vi "reward_behavior_timeout_9s_probes_opto_2-5s_ISI.vi"() -> ()   [LabVIEW 2019]
doc: "The myRIO Project template acquires acceleration data from the onboard accelerometer and displays the changes of acceleration values in a waveform chart."
uses:
  <vilib>/Analysis/Matrix/Datatypes/RealMatrix.ctl
  <vilib>/myRIO/Common/Instrument Driver Framework/myRIO v1.0/Encoder/typedefs/Encoder Signal Mode.ctl
  <vilib>/myRIO/Instrument Drivers/Onboard IO/Encoder/typedefs/Encoder Reference.ctl
  <vilib>/myRIO/Common/Instrument Driver Framework/Utilities/typedefs/myRIO Generic Hardware Reference.ctl
  <vilib>/myRIO/Common/Instrument Driver Framework/Utilities/typedefs/Hardware Version Enum.ctl
  <vilib>/myRIO/Common/Instrument Driver Framework/Utilities/typedefs/myRIO v1.0 Reference.ctl
  <vilib>/myRIO/Common/Instrument Driver Framework/Utilities/typedefs/Generic FPGA Reference.ctl
  <vilib>/myRIO/Common/Instrument Driver Framework/myRIO v1.0/Encoder/typedefs/Encoder Channels Enum.ctl
  <vilib>/myRIO/Common/Instrument Driver Framework/myRIO v1.0/Encoder/typedefs/Encoder Configuration v1.0.ctl
  <vilib>/userdefined/High Color/nirio_resource_hc.ctl
  <vilib>/myRIO/Instrument Drivers/Onboard IO/DIO/typedefs/DIO Reference.ctl
  <vilib>/myRIO/Common/Instrument Driver Framework/myRIO v1.0/DIO/typedefs/DIO Channels List.ctl
  <vilib>/myRIO/Common/Instrument Driver Framework/myRIO v1.0/DIO/typedefs/DIO Channels Enum.ctl
  <vilib>/myRIO/Common/Instrument Driver Framework/Utilities/vis/Is FPGA Ref Available.vi
  <vilib>/myRIO/Common/Instrument Driver Framework/myRIO v1.0/Encoder/vis/myRIO v1.1 Open Encoder.vi
  <vilib>/myRIO/Instrument Drivers/Onboard IO/Encoder/vis/Read.vi
  <vilib>/myRIO/Common/Instrument Driver Framework/myRIO v1.0/DIO/vis/myRIO v1.1 Open DIO.vi
  <vilib>/myRIO/Instrument Drivers/Onboard IO/DIO/vis/Write.vi
  <vilib>/myRIO/Instrument Drivers/Onboard IO/DIO/vis/Read.vi
  <vilib>/myRIO/Common/Instrument Driver Framework/Utilities/vis/Validate Channels.vi
  <vilib>/myRIO/Common/Instrument Driver Framework/myRIO v1.0/Encoder/vis/myRIO v1.0 Reserve Encoder.vi
  <vilib>/myRIO/Common/Instrument Driver Framework/myRIO v1.0/DIO/vis/myRIO v1.0 Reserve DIO.vi
  <vilib>/myRIO/Common/Instrument Driver Framework/myRIO v1.0/Encoder/vis/myRIO v1.0 Build MUX Configuration Encoder.vi
  <vilib>/myRIO/Common/Instrument Driver Framework/myRIO v1.0/Resource Manager/vis/myRIO v1.0 Reserve Channel List.vi
  <vilib>/myRIO/Common/Instrument Driver Framework/myRIO v1.0/DIO/vis/myRIO v1.0 Build MUX Configuration DIO.vi
  <vilib>/myRIO/Common/Instrument Driver Framework/myRIO v1.0/Resource Manager/vis/myRIO v1.0 Create Configuration List.vi
  <vilib>/myRIO/Common/Instrument Driver Framework/myRIO v1.0/Resource Manager/vis/myRIO v1.0 Reserve Channel.vi
  <vilib>/myRIO/Common/Instrument Driver Framework/myRIO v1.0/Resource Manager/vis/myRIO v1.0 Unreserve Channel.vi
  <vilib>/myRIO/Common/Instrument Driver Framework/myRIO v1.0/Resource Manager/vis/myRIO v1.0 Build Mutex Name.vi
  <vilib>/Utility/VariantDataType/GetNumericInfo.vi
  <vilib>/Utility/error.llb/Error Cluster From Error Code.vi
  <vilib>/myRIO/Common/Instrument Driver Framework/myRIO v1.0/myRIO v1.1 Open.vi
  <vilib>/myRIO/Common/Instrument Driver Framework/Utilities/vis/IO Manager.vi
  <vilib>/myRIO/Common/Instrument Driver Framework/Utilities/vis/Configuration Manager.vi
  <vilib>/myRIO/Common/Instrument Driver Framework/myRIO v1.0/Resource Manager/vis/myRIO v1.0 Configure IO.vi
  <vilib>/myRIO/Common/Instrument Driver Framework/myRIO v1.0/myRIO v1.0 Close.vi
  <vilib>/myRIO/Common/Instrument Driver Framework/myRIO v1.0/Encoder/vis/myRIO v1.0 Configure Encoder.vi
  <vilib>/myRIO/Common/Instrument Driver Framework/myRIO v1.0/Encoder/vis/myRIO v1.0 Read Encoder.vi
  <vilib>/myRIO/Common/Instrument Driver Framework/myRIO v1.0/DIO/vis/myRIO v1.0 Read DIO.vi
  <vilib>/myRIO/Common/Instrument Driver Framework/myRIO v1.0/DIO/vis/myRIO v1.0 Write DIO.vi
  <vilib>/myRIO/Express VI/Onboard IO/Encoder/Encoder Express VI.xnode
  <vilib>/myRIO/Instrument Drivers/Onboard IO/Encoder/vis/myRIO Encoder Open.xnode
  <vilib>/myRIO/Express VI/Onboard IO/DI/DI Express VI.xnode
  <vilib>/myRIO/Instrument Drivers/Onboard IO/DIO/vis/myRIO DIO Open.xnode
  <vilib>/myRIO/Express VI/Onboard IO/DO/DO Express VI.xnode
  <vilib>/myRIO/Instrument Drivers/Onboard IO/Encoder/Encoder.lvlib
  <vilib>/myRIO/Instrument Drivers/Onboard IO/DIO/DIO.lvlib
  <vilib>/Analysis/Matrix/NI_Matrix.lvlib
panel:
  out "Timings":dbl[](array[numeric])
  out "ISI":dbl
  out "ISI start time":dbl
  out "Time_out":bool=TRUE
  out "Time since lick":dbl
  out "Time of last lick":dbl
  out "Rewarded trials":dbl[](array[numeric])
  out "Rewards":u16
  out "Active Trial":bool
  out "Array temp2":T1
  out "Stimuli Loaded":bool
  out "Stim_ID":dbl[](array[numeric])
  out "Reward_mat":dbl[](array[numeric])
  out "Reward":bool=TRUE
  out "Frame clock":i32
  out "Licks":u32
  out "Lick":bool
  out "Time":dbl
  out "Stop":bool
  in  "Frames to collect":u32
  out "Overflow?":bool
  out "Counter Value":i32
  out "Velocity":dbl
  out "Velocity Plot":dbl[](graph)
  out "Velocity array":dbl[](array[numeric])
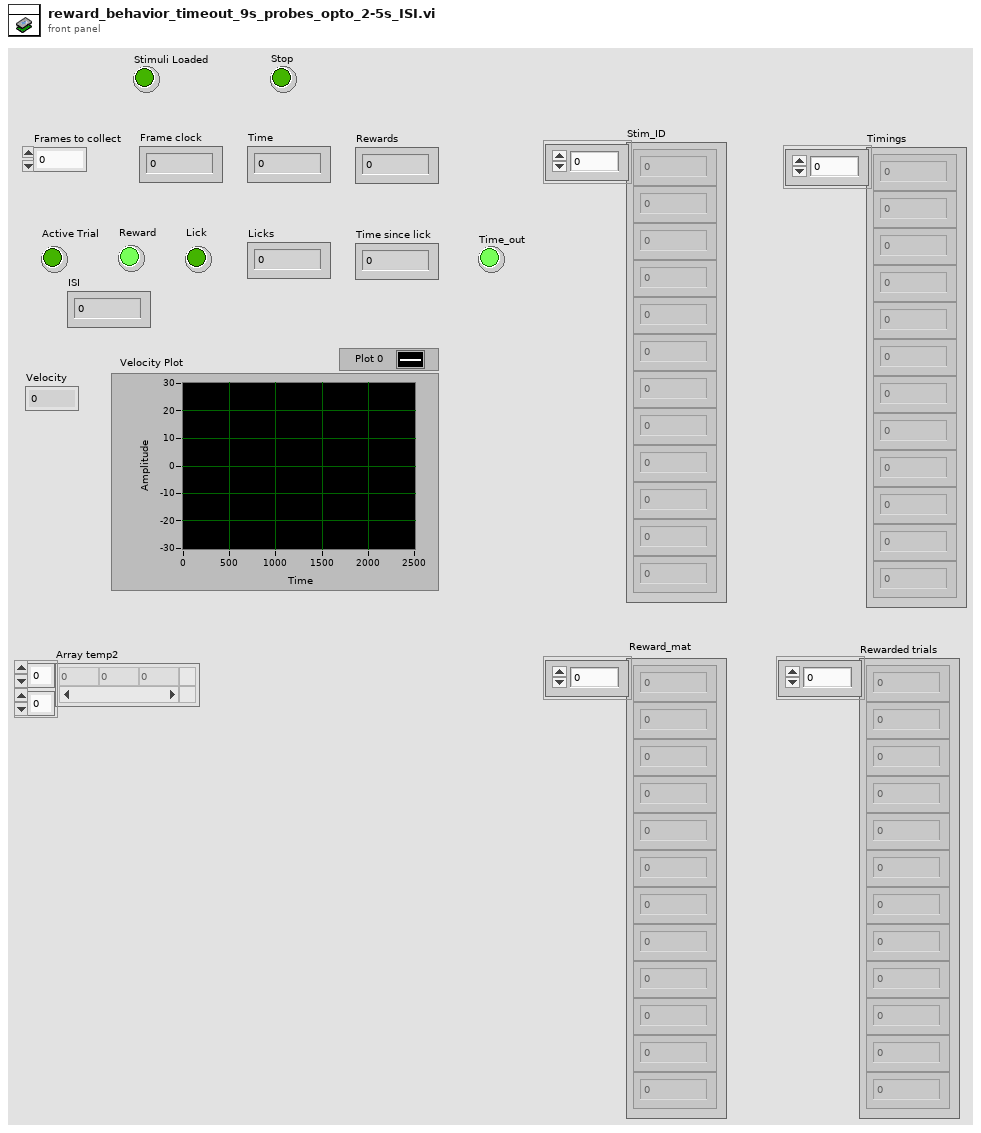
[diagram p1: front panel]
types:
  T1 = typedef "NI_Matrix.lvlib/RealMatrix.ctl" = dbl[][]
  T2 = typedef "Encoder.lvlib/Encoder Reference.ctl" = cluster{"myRIO Reference":T3, "Encoder Channels Enum":T7}
  T3 = typedef "myRIO Generic Hardware Reference.ctl" = cluster{"myRIO Model":T4, "myRIO Hardware Reference":T5}
  T4 = typedef "Hardware Version Enum.ctl" = enum16{"Unknown", "myRIO-1900", "myRIO-1950", "roboRIO", "NI ELVIS RIO CM", "ELVIS III"}
  T5 = typedef "myRIO v1.0 Reference.ctl" = cluster{"Generic FPGA Reference":T6, "Allow multiple opens":bool}
  T6 = typedef "Generic FPGA Reference.ctl" = refnum<k20>
  T7 = typedef "Encoder Channels Enum.ctl" = enum16{"Not Connected", "C/ENC0", "C/ENC1", "A/ENC", "A/ENC0", "A/ENC1", "A/ENC2", "A/ENC3", "A/ENC4", "A/ENC5", "A/ENC6", "A/ENC7", "A/ENC8", "A/ENC9", "B/ENC", "B/ENC0", "B/ENC1", "B/ENC2", "B/ENC3", "B/ENC4", "B/ENC5", "B/ENC6", "B/ENC7", "B/ENC8", "B/ENC9", "DIO/ENC0", "DIO/ENC1", "DIO/ENC2", "DIO/ENC3", "DIO/ENC4"}
  T8 = typedef "Encoder Signal Mode.ctl" = enum16{"Quadrature phase signal", "Step and direction signal"}
  T9 = typedef "nirio_resource_hc.ctl" = tag
  T10 = typedef "DIO.lvlib/DIO Reference.ctl" = cluster{"myRIO Reference":T3, "DIO Channels List":T11}
  T11 = typedef "DIO Channels List.ctl" = T12[]
  T12 = typedef "DIO Channels Enum.ctl" = enum16{"Not Connected", "C/DIO0", "C/DIO1", "C/DIO2", "C/DIO3", "C/DIO4", "C/DIO5", "C/DIO6", "C/DIO7", "A/DIO0", "A/DIO1", "A/DIO2", "A/DIO3", "A/DIO4", "A/DIO5", "A/DIO6", "A/DIO7", "A/DIO8", "A/DIO9", "A/DIO10", "A/DIO11", "A/DIO12", "A/DIO13", "A/DIO14", "A/DIO15", "A/DIO16", "A/DIO17", "A/DIO18", "A/DIO19", "B/DIO0", "B/DIO1", "B/DIO2", "B/DIO3", "B/DIO4", "B/DIO5", "B/DIO6", "B/DIO7", "B/DIO8", "B/DIO9", "B/DIO10", "B/DIO11", "B/DIO12", "B/DIO13", "B/DIO14", "B/DIO15", "B/DIO16", "B/DIO17", "B/DIO18", "B/DIO19", "LED0", "LED1", "LED2", "LED3", "Button0", "DIO/DIO0", "DIO/DIO1", "DIO/DIO2", "DIO/DIO3", "DIO/DIO4", "DIO/DIO5", "DIO/DIO6", "DIO/DIO7", "DIO/DIO8", "DIO/DIO9", "SPI/CS0", "SPI/CS1", "SPI/CS2", "SPI/CS3", "LED RADIO (Green)", "LED RADIO (Red)", "LED COMM (Green)", "LED COMM (Red)", "LED MODE (Green)", "LED MODE (Red)"}
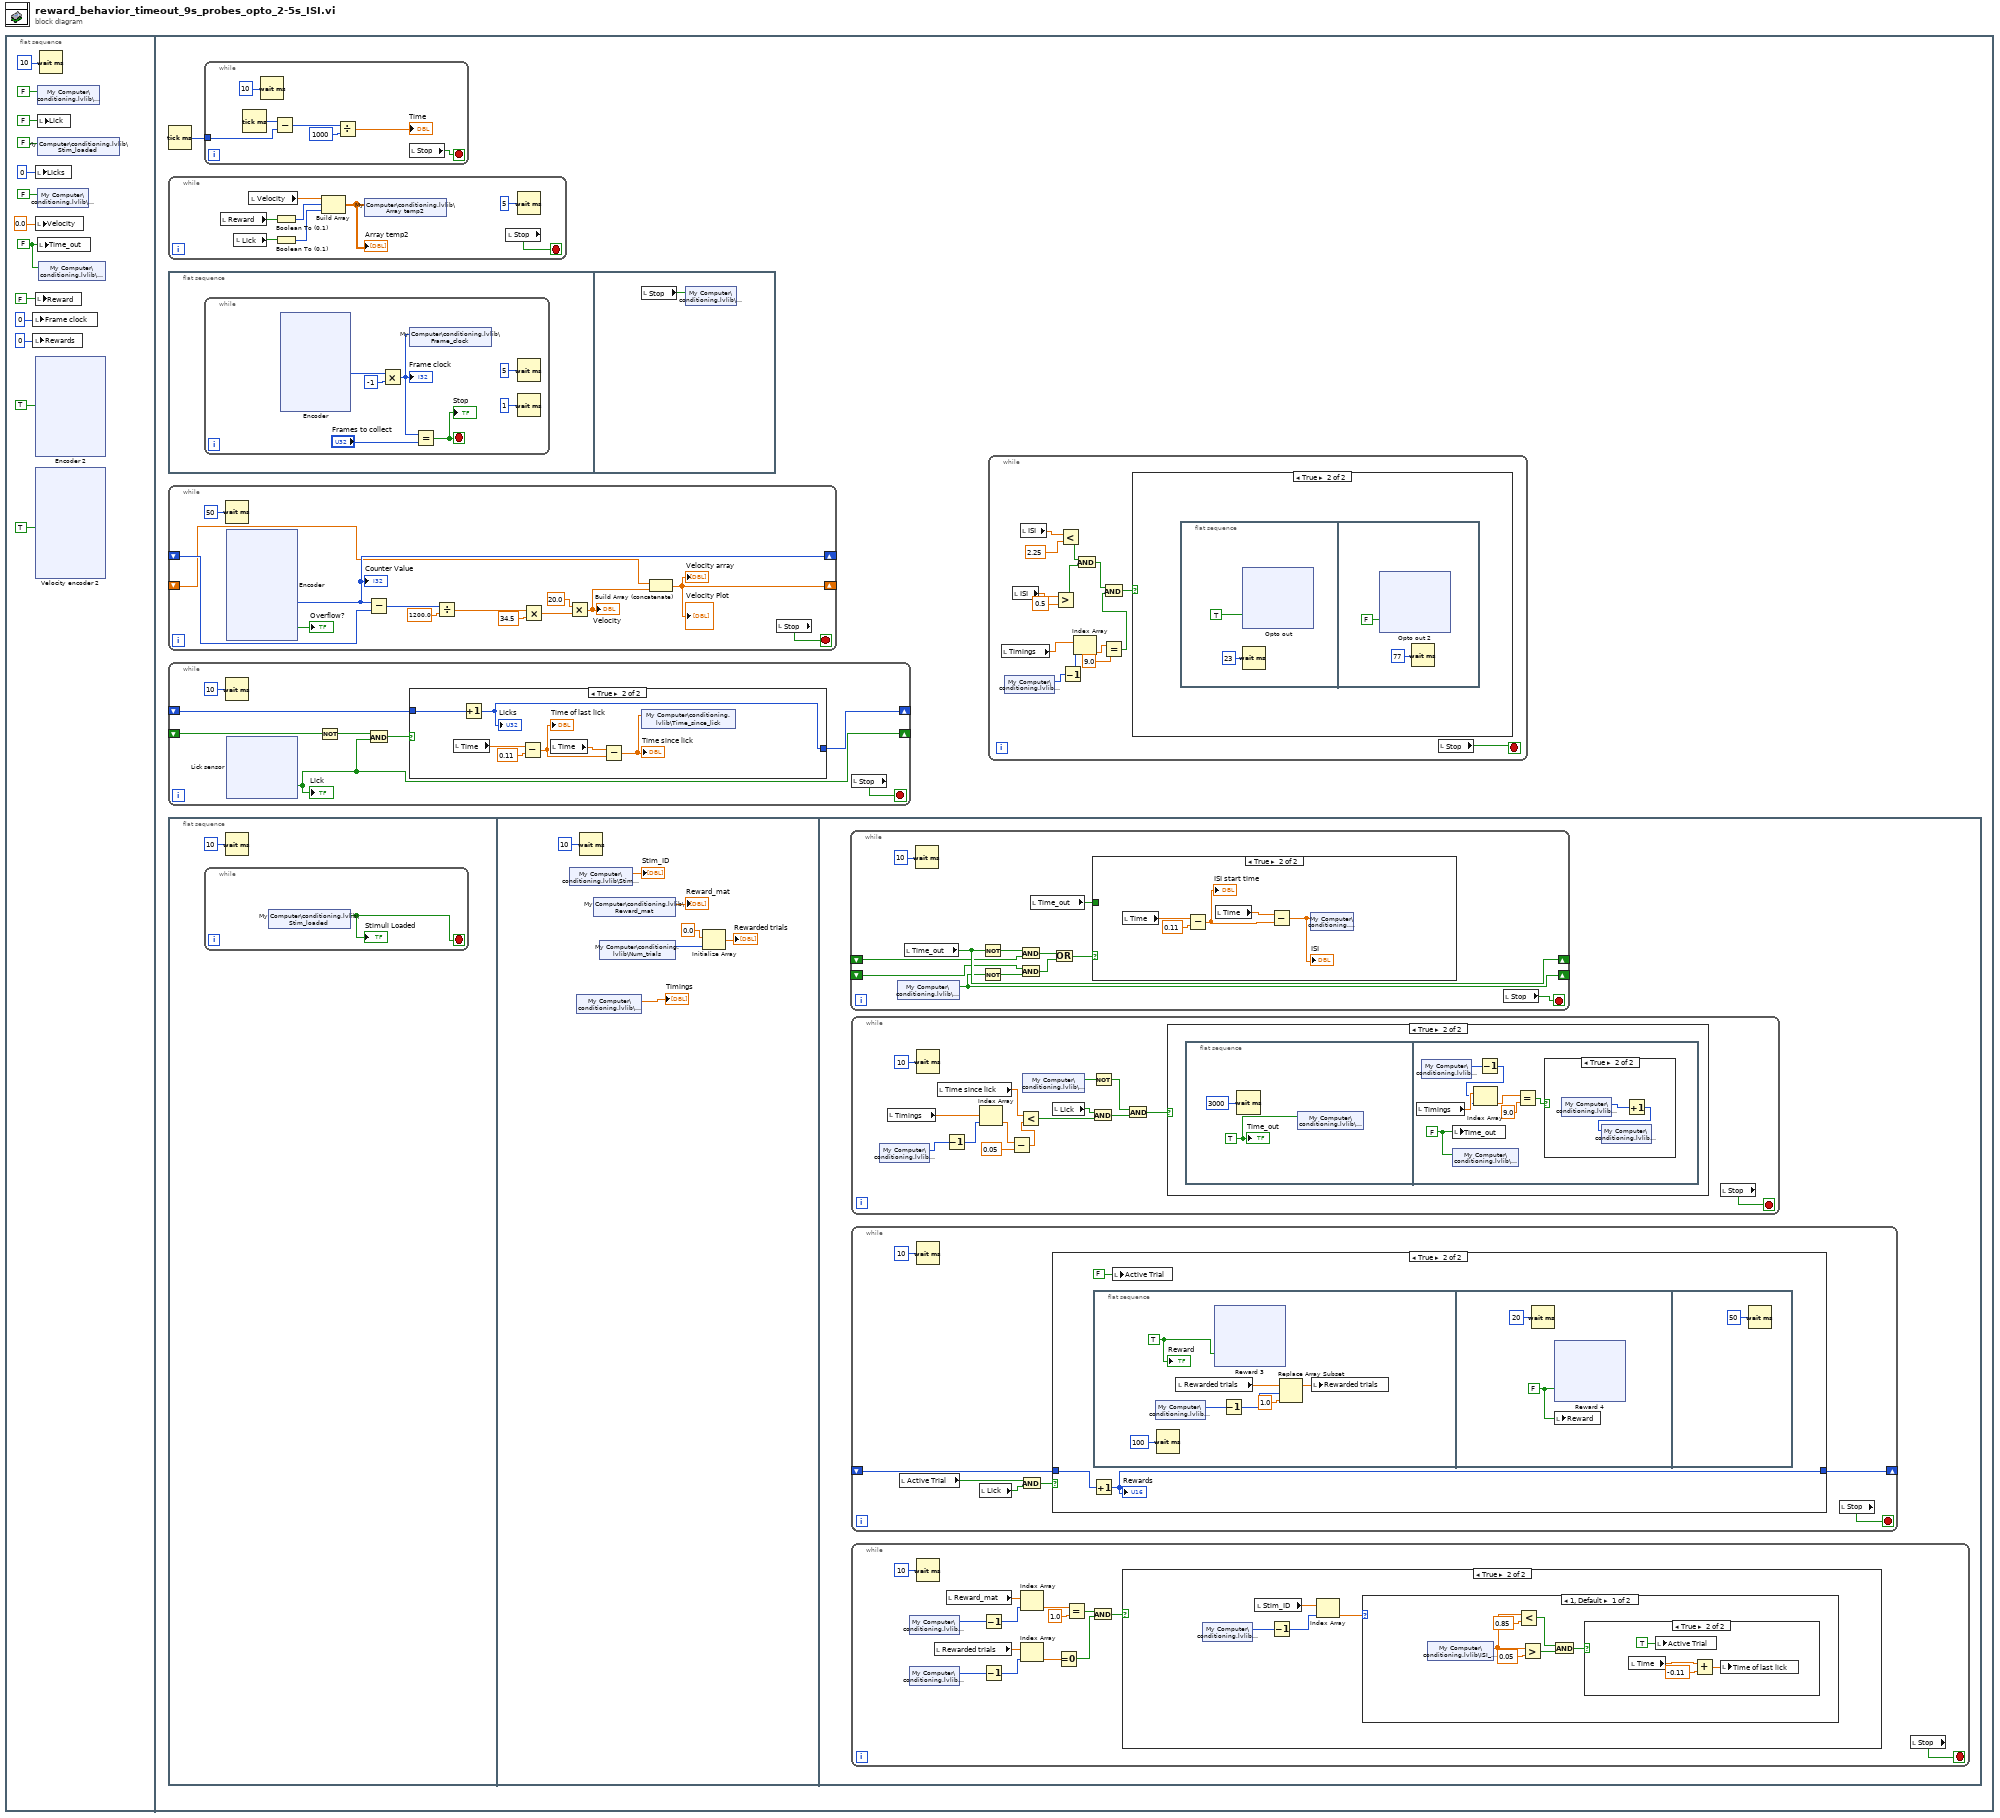
[diagram p0: block diagram]
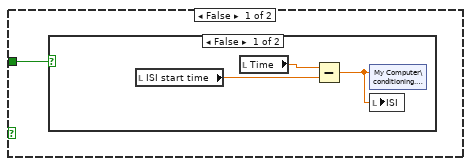
[diagram p5: hidden frame]
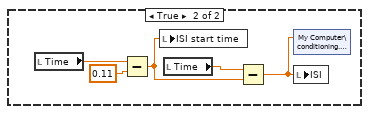
[diagram p6: hidden frame]
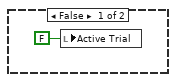
[diagram p7: hidden frame]
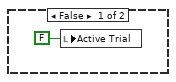
[diagram p8: hidden frame]
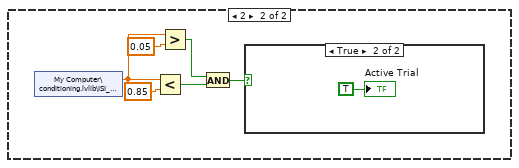
[diagram p9: hidden frame]
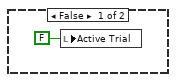
[diagram p10: hidden frame]
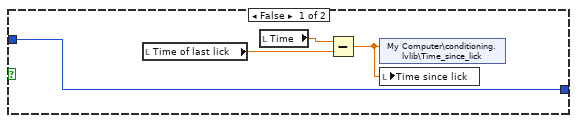
[diagram p12: hidden frame]
diagram:
  n1 = flat-sequence {
    frame #0 {
      w1 = FALSE ("Time_out")
      n2 = local write "Frame clock"(u32 0 ("Frames")) -> ()
      n3 = local write "Rewards"(u16 0 ("Rewards")) -> ()
      n4 = local write "Licks"(u32 0 ("Licks")) -> ()
      n5 = local write "Velocity"(0.0 ("Velocity")) -> ()
      n6 = local write "Reward"(FALSE ("Give reward")) -> ()
      n7 = xnode "Encoder 2"("Reset Counter"=TRUE) -> ()  [unwired: 1 in, 4 out]
      n8 = xnode "Velocity encoder 2"("Reset Counter"=TRUE) -> ()  [unwired: 1 in, 4 out]
      n9 = shared-variable "My Computer\\conditioning.lvlib\\Display"(FALSE ("Display")) -> ()  [unwired: 1 in, 1 out]
      n10 = local write "Lick"(FALSE ("Lick")) -> ()
      n11 = shared-variable "My Computer\\conditioning.lvlib\\Stim_loaded"(FALSE ("Stim_loaded")) -> ()  [unwired: 1 in, 1 out]
      n12 = shared-variable "My Computer\\conditioning.lvlib\\Stop"(FALSE ("Stop")) -> ()  [unwired: 1 in, 1 out]
      n13 = local write "Time_out"(w1) -> ()
      n14 = shared-variable "My Computer\\conditioning.lvlib\\Timeout"(w1) -> ()  [unwired: 1 in, 1 out]
      n15 = Wait (ms)(milliseconds to wait=u32 10) -> ()  [unwired: 1 out]
    }
    frame #1 {
      n16 = Tick Count (ms)() -> (millisecond timer value=w106:u32)
      n17 = while {
        stop <- w197 stop-if-true
        n18 = local read "Reward"() -> (w202:bool)
        n19 = local read "Lick"() -> (w203:bool)
        n20 = local read "Velocity"() -> (w201:dbl)
        n21 = Boolean To (0,1)(Boolean=w202) -> (0, 1=w200:i16)
        n22 = Boolean To (0,1)(Boolean=w203) -> (0, 1=w199:i16)
        n23 = Build Array(w201, w200, w199) -> (w196:T1)
        "Array temp2" <- w196
        n24 = shared-variable "My Computer\\conditioning.lvlib\\Array temp2"(w196) -> ()  [unwired: 1 in, 1 out]
        n25 = local read "Stop"() -> (w197:bool)
        n26 = Wait (ms)(milliseconds to wait=u32 5) -> ()  [unwired: 1 out]
      }
      n27 = flat-sequence {
        frame #0 {
          n28 = while {
            stop <- w395 stop-if-true
            n29 = xnode "Encoder"() -> ("Counter Value"=w399:i32)  [unwired: 2 in, 3 out]
            n30 = Multiply(x=w399, y=-1) -> (x*y=w394:i32)
            "Frame clock" <- w394
            n31 = shared-variable "My Computer\\conditioning.lvlib\\Frame_clock"(w394) -> ()  [unwired: 1 in, 1 out]
            n32 = Equal?(x=w394, y="Frames to collect") -> (x = y?=w395:bool)
            "Stop" <- w395
            n33 = Wait (ms)(milliseconds to wait=u32 5) -> ()  [unwired: 1 out]
            n34 = Wait (ms)(milliseconds to wait=u32 1) -> ()  [unwired: 1 out]
          }
        }
        frame #1 {
          n35 = local read "Stop"() -> (w447:bool)
          n36 = shared-variable "My Computer\\conditioning.lvlib\\Stop"(w447) -> ()  [unwired: 1 in, 1 out]
        }
      }
      n37 = while {
        shift-right: [w512] -> _
        shift-left: _ -> [w513]
        shift-right: [w504] -> _
        shift-left: _ -> [w503]
        stop <- w502 stop-if-true
        n38 = Wait (ms)(milliseconds to wait=u32 50) -> ()  [unwired: 1 out]
        n39 = xnode "Encoder"() -> ("Counter Value"=w512:i32, "Overflow?"=→"Overflow?":bool)  [unwired: 2 in, 2 out]
        "Counter Value" <- w512
        n40 = Subtract(x=w512, y=w513) -> (x-y=w505:i32)
        n41 = Divide(x=w505, y=1200.0 ("600")) -> (x/y=w510:dbl)
        n42 = Multiply(x=w510, y=34.5) -> (x*y=w508:dbl)
        n43 = Multiply(x=20.0, y=w508) -> (x*y=w506:dbl)
        "Velocity" <- w506
        n44 = Build Array (concatenate)(w503, w506) -> (w504:dbl[])
        "Velocity Plot" <- w504
        "Velocity array" <- w504
        n45 = local read "Stop"() -> (w502:bool)
      }
      n46 = while {
        shift-right: [w454] -> _
        shift-left: _ -> [w453]
        shift-right: [w448] -> _
        shift-left: _ -> [w451]
        stop <- w452 stop-if-true
        n47 = Wait (ms)(milliseconds to wait=u32 10) -> ()  [unwired: 1 out]
        n48 = xnode "Lick sensor"() -> ("C/DIO1 (DIO1)"=w448:bool)  [unwired: 1 in, 1 out]
        "Lick" <- w448
        n49 = Not(x=w451) -> (.not. x?=w450:bool)
        n50 = And(x=w450, y=w448) -> (x .and. y?=w449:bool)
        n51 = case shown="True" w449 {
          tunnel: [w459 w466] -> w454
          tunnel: w453 -> [w459 w465]
          frame False {
            n52 = local read "Time of last lick"() -> (w457:dbl)
            n53 = local read "Time"() -> (w458:dbl)
            n54 = Subtract(x=w458, y=w457) -> (x-y=w456:dbl)
            n55 = shared-variable "My Computer\\conditioning.lvlib\\Time_since_lick"(w456) -> ()  [unwired: 1 in, 1 out]
            n56 = local write "Time since lick"(w456) -> ()
          }
          frame True {
            n57 = local read "Time"() -> (w462:dbl)
            n58 = Increment(x=w465) -> (x+1=w466:u32)
            "Licks" <- w466
            n59 = Subtract(x=w462, y=0.11) -> (x-y=w460:dbl)
            "Time of last lick" <- w460
            n60 = local read "Time"() -> (w464:dbl)
            n61 = Subtract(x=w464, y=w460) -> (x-y=w463:dbl)
            "Time since lick" <- w463
            n62 = shared-variable "My Computer\\conditioning.lvlib\\Time_since_lick"(w463) -> ()  [unwired: 1 in, 1 out]
          }
        }
        n63 = local read "Stop"() -> (w452:bool)
      }
      n64 = flat-sequence {
        frame #0 {
          n65 = while {
            stop <- w205 stop-if-true
            n66 = shared-variable "My Computer\\conditioning.lvlib\\Stim_loaded"() -> (w205:bool)  [unwired: 1 in, 1 out]
            "Stimuli Loaded" <- w205
          }
          n67 = Wait (ms)(milliseconds to wait=u32 10) -> ()  [unwired: 1 out]
        }
        frame #1 {
          n68 = shared-variable "My Computer\\conditioning.lvlib\\Stim_ID"() -> (→"Stim_ID":dbl[])  [unwired: 1 in, 1 out]
          n69 = shared-variable "My Computer\\conditioning.lvlib\\Timings"() -> (→"Timings":dbl[])  [unwired: 1 in, 1 out]
          n70 = Wait (ms)(milliseconds to wait=u32 10) -> ()  [unwired: 1 out]
          n71 = shared-variable "My Computer\\conditioning.lvlib\\Reward_mat"() -> (→"Reward_mat":dbl[])  [unwired: 1 in, 1 out]
          n72 = shared-variable "My Computer\\conditioning.lvlib\\Num_trials"() -> (w209:u32)  [unwired: 1 in, 1 out]
          n73 = Initialize Array(0.0 ("element"), w209) -> (→"Rewarded trials":dbl[])
        }
        frame #2 {
          n74 = while {
            shift-right: [w249] -> _
            shift-left: _ -> [w247]
            shift-right: [w245] -> _
            shift-left: _ -> [w244]
            stop <- w250 stop-if-true
            n75 = shared-variable "My Computer\\conditioning.lvlib\\Display"() -> (w245:bool)  [unwired: 1 in, 1 out]
            n76 = local read "Time_out"() -> (w249:bool)
            n77 = Wait (ms)(milliseconds to wait=u32 10) -> ()  [unwired: 1 out]
            n78 = Not(x=w249) -> (.not. x?=w248:bool)
            n79 = Not(x=w245) -> (.not. x?=w243:bool)
            n80 = And(x=w248, y=w247) -> (x .and. y?=w242:bool)
            n81 = And(x=w244, y=w243) -> (x .and. y?=w241:bool)
            n82 = local read "Time_out"() -> (w246:bool)
            n83 = Or(x=w242, y=w241) -> (x .or. y?=w240:bool)
            n84 = case shown="True" w240 {
              tunnel: w246 -> [w251 _]
              frame False {
                n85 = case shown="False" w251 {
                  frame False {
                    n86 = local read "ISI start time"() -> (w254:dbl)
                    n87 = local read "Time"() -> (w253:dbl)
                    n88 = Subtract(x=w253, y=w254) -> (x-y=w252:dbl)
                    n89 = shared-variable "My Computer\\conditioning.lvlib\\ISI"(w252) -> ()  [unwired: 1 in, 1 out]
                    n90 = local write "ISI"(w252) -> ()
                  }
                  frame True {
                    n91 = local read "Time"() -> (w259:dbl)
                    n92 = Subtract(x=w259, y=0.11) -> (x-y=w256:dbl)
                    n93 = local write "ISI start time"(w256) -> ()
                    n94 = local read "Time"() -> (w257:dbl)
                    n95 = Subtract(x=w257, y=w256) -> (x-y=w255:dbl)
                    n96 = shared-variable "My Computer\\conditioning.lvlib\\ISI"(w255) -> ()  [unwired: 1 in, 1 out]
                    n97 = local write "ISI"(w255) -> ()
                  }
                }
              }
              frame True {
                n98 = local read "Time"() -> (w264:dbl)
                n99 = Subtract(x=w264, y=0.11) -> (x-y=w261:dbl)
                "ISI start time" <- w261
                n100 = local read "Time"() -> (w262:dbl)
                n101 = Subtract(x=w262, y=w261) -> (x-y=w260:dbl)
                "ISI" <- w260
                n102 = shared-variable "My Computer\\conditioning.lvlib\\ISI"(w260) -> ()  [unwired: 1 in, 1 out]
              }
            }
            n103 = local read "Stop"() -> (w250:bool)
          }
          n104 = while {
            stop <- w227 stop-if-true
            n105 = shared-variable "My Computer\\conditioning.lvlib\\Trial"() -> (w217:u32)  [unwired: 1 in, 1 out]
            n106 = local read "Timings"() -> (w218:dbl[])
            n107 = Wait (ms)(milliseconds to wait=u32 10) -> ()  [unwired: 1 out]
            n108 = local read "Time since lick"() -> (w226:dbl)
            n109 = Decrement(x=w217) -> (x-1=w216:u32)
            n110 = Index Array(array=w218, index=w216) -> (element=w215:dbl)
            n111 = Subtract(x=w215, y=0.05) -> (x-y=w213:dbl)
            n112 = Less?(x=w226, y=w213) -> (x < y?=w225:bool)
            n113 = shared-variable "My Computer\\conditioning.lvlib\\Display"() -> (w222:bool)  [unwired: 1 in, 1 out]
            n114 = local read "Lick"() -> (w224:bool)
            n115 = Not(x=w222) -> (.not. x?=w221:bool)
            n116 = And(x=w224, y=w225) -> (x .and. y?=w220:bool)
            n117 = And(x=w221, y=w220) -> (x .and. y?=w219:bool)
            n118 = case shown="True" w219 {
              frame False {
              }
              frame True {
                n119 = flat-sequence {
                  frame #0 {
                    w229 = TRUE
                    n120 = Wait (ms)(milliseconds to wait=u32 3000) -> ()  [unwired: 1 out]
                    n121 = shared-variable "My Computer\\conditioning.lvlib\\Timeout"(w229) -> ()  [unwired: 1 in, 1 out]
                    "Time_out" <- w229
                  }
                  frame #1 {
                    w236 = FALSE ("Timeout")
                    n122 = local read "Timings"() -> (w235:dbl[])
                    n123 = shared-variable "My Computer\\conditioning.lvlib\\Trial"() -> (w231:u32)  [unwired: 1 in, 1 out]
                    n124 = local write "Time_out"(w236) -> ()
                    n125 = shared-variable "My Computer\\conditioning.lvlib\\Timeout"(w236) -> ()  [unwired: 1 in, 1 out]
                    n126 = Decrement(x=w231) -> (x-1=w230:u32)
                    n127 = Index Array(array=w235, index=w230) -> (element=w233:dbl)
                    n128 = Equal?(x=w233, y=9.0) -> (x = y?=w234:bool)
                    n129 = case shown="True" w234 {
                      frame False {
                      }
                      frame True {
                        n130 = shared-variable "My Computer\\conditioning.lvlib\\Trial"() -> (w238:u32)  [unwired: 1 in, 1 out]
                        n131 = Increment(x=w238) -> (x+1=w237:u32)
                        n132 = shared-variable "My Computer\\conditioning.lvlib\\Trial"(w237) -> ()  [unwired: 1 in, 1 out]
                      }
                    }
                  }
                }
              }
            }
            n133 = local read "Stop"() -> (w227:bool)
          }
          n134 = while {
            shift-right: [w306] -> _
            shift-left: _ -> [w305]
            stop <- w309 stop-if-true
            n135 = local read "Active Trial"() -> (w303:bool)
            n136 = Wait (ms)(milliseconds to wait=u32 10) -> ()  [unwired: 1 out]
            n137 = local read "Lick"() -> (w304:bool)
            n138 = And(x=w303, y=w304) -> (x .and. y?=w307:bool)
            n139 = case shown="True" w307 {
              tunnel: [w310 w313] -> w306
              tunnel: w305 -> [w310 w312]
              frame False {
              }
              frame True {
                n140 = Increment(x=w312) -> (x+1=w313:u16)
                "Rewards" <- w313
                n141 = flat-sequence {
                  frame #0 {
                    w319 = TRUE ("C/DIO0 (DIO0)")
                    n142 = shared-variable "My Computer\\conditioning.lvlib\\Trial"() -> (w318:u32)  [unwired: 1 in, 1 out]
                    n143 = Wait (ms)(milliseconds to wait=u32 100) -> ()  [unwired: 1 out]
                    n144 = local read "Rewarded trials"() -> (w316:dbl[])
                    n145 = xnode "Reward 3"("C/DIO0 (DIO0)"=w319) -> ()  [unwired: 1 in, 1 out]
                    n146 = Decrement(x=w318) -> (x-1=w317:u32)
                    n147 = Replace Array Subset(array=w316, new element=1.0 ("new element/subarray"), index=w317) -> (w314:dbl[])
                    n148 = local write "Rewarded trials"(w314) -> ()
                    "Reward" <- w319
                  }
                  frame #1 {
                    w357 = FALSE ("C/DIO0 (DIO0)")
                    n149 = Wait (ms)(milliseconds to wait=u32 20) -> ()  [unwired: 1 out]
                    n150 = xnode "Reward 4"("C/DIO0 (DIO0)"=w357) -> ()  [unwired: 1 in, 1 out]
                    n151 = local write "Reward"(w357) -> ()
                  }
                  frame #2 {
                    n152 = Wait (ms)(milliseconds to wait=u32 50) -> ()  [unwired: 1 out]
                  }
                }
                n153 = local write "Active Trial"(FALSE ("Active Trial")) -> ()
              }
            }
            n154 = local read "Stop"() -> (w309:bool)
          }
          n155 = while {
            stop <- w278 stop-if-true
            n156 = shared-variable "My Computer\\conditioning.lvlib\\Trial"() -> (w274:u32)  [unwired: 1 in, 1 out]
            n157 = shared-variable "My Computer\\conditioning.lvlib\\Trial"() -> (w270:u32)  [unwired: 1 in, 1 out]
            n158 = Wait (ms)(milliseconds to wait=u32 10) -> ()  [unwired: 1 out]
            n159 = local read "Rewarded trials"() -> (w271:dbl[])
            n160 = local read "Reward_mat"() -> (w273:dbl[])
            n161 = Decrement(x=w274) -> (x-1=w275:u32)
            n162 = Decrement(x=w270) -> (x-1=w269:u32)
            n163 = Index Array(array=w273, index=w275) -> (element=w276:dbl)
            n164 = Index Array(array=w271, index=w269) -> (element=w268:dbl)
            n165 = Equal To 0?(x=w268) -> (x = 0?=w267:bool)
            n166 = Equal?(x=w276, y=1.0) -> (x = y?=w266:bool)
            n167 = And(x=w266, y=w267) -> (x .and. y?=w265:bool)
            n168 = case shown="True" w265 {
              frame False {
                n169 = local write "Active Trial"(FALSE ("Active_trial")) -> ()
              }
              frame True {
                n170 = shared-variable "My Computer\\conditioning.lvlib\\Trial"() -> (w281:u32)  [unwired: 1 in, 1 out]
                n171 = local read "Stim_ID"() -> (w283:dbl[])
                n172 = Decrement(x=w281) -> (x-1=w282:u32)
                n173 = Index Array(array=w283, index=w282) -> (element=w280:dbl)
                n174 = case shown="1, Default" w280 {
                  frame 1, Default {
                    n175 = shared-variable "My Computer\\conditioning.lvlib\\ISI_Time"() -> (w288:dbl)  [unwired: 1 in, 1 out]
                    n176 = Less?(x=w288, y=0.85) -> (x < y?=w286:bool)
                    n177 = Greater?(x=w288, y=0.05) -> (0:w285:bool)
                    n178 = And(x=w286, y=w285) -> (x .and. y?=w284:bool)
                    n179 = case shown="True" w284 {
                      frame False {
                        n180 = local write "Active Trial"(FALSE ("Active Trial")) -> ()
                      }
                      frame True {
                        n181 = local read "Time"() -> (w293:dbl)
                        n182 = local write "Active Trial"(TRUE ("Active Trial")) -> ()
                        n183 = Add(x=w293, y=-0.11) -> (x+y=w291:dbl)
                        n184 = local write "Time of last lick"(w291) -> ()
                      }
                    }
                  }
                  frame 2 {
                    n185 = shared-variable "My Computer\\conditioning.lvlib\\ISI_Time"() -> (w299:dbl)  [unwired: 1 in, 1 out]
                    n186 = Less?(x=w299, y=0.85) -> (x < y?=w296:bool)
                    n187 = Greater?(x=w299, y=0.05) -> (0:w297:bool)
                    n188 = And(x=w297, y=w296) -> (x .and. y?=w295:bool)
                    n189 = case shown="True" w295 {
                      frame False {
                        n190 = local write "Active Trial"(FALSE ("Active Trial")) -> ()
                      }
                      frame True {
                        "Active Trial" <- TRUE ("Active Trial")
                      }
                    }
                  }
                }
              }
            }
            n191 = local read "Stop"() -> (w278:bool)
          }
        }
      }
      n192 = while {
        tunnel: w106 -> [w567]
        stop <- w565 stop-if-true
        n193 = Tick Count (ms)() -> (millisecond timer value=w568:u32)
        n194 = Wait (ms)(milliseconds to wait=u32 10) -> ()  [unwired: 1 out]
        n195 = Subtract(x=w568, y=w567) -> (x-y=w564:u32)
        n196 = Divide(x=w564, y=u32 1000) -> (x/y=→"Time":dbl)
        n197 = local read "Stop"() -> (w565:bool)
      }
      n198 = while {
        stop <- w107 stop-if-true
        n199 = local read "Timings"() -> (w113:dbl[])
        n200 = shared-variable "My Computer\\conditioning.lvlib\\Trial"() -> (w115:u32)  [unwired: 1 in, 1 out]
        n201 = local read "ISI"() -> (w118:dbl)
        n202 = local read "ISI"() -> (w121:dbl)
        n203 = Greater?(x=w118, y=0.5) -> (0:w116:bool)
        n204 = Less?(x=w121, y=2.25) -> (x < y?=w119:bool)
        n205 = Decrement(x=w115) -> (x-1=w114:u32)
        n206 = Index Array(array=w113, index=w114) -> (element=w112:dbl)
        n207 = And(x=w119, y=w116) -> (x .and. y?=w108:bool)
        n208 = Equal?(x=w112, y=9.0) -> (x = y?=w109:bool)
        n209 = And(x=w108, y=w109) -> (x .and. y?=w110:bool)
        n210 = case shown="True" w110 {
          frame False {
          }
          frame True {
            n211 = flat-sequence {
              frame #0 {
                n212 = Wait (ms)(milliseconds to wait=u32 23) -> ()  [unwired: 1 out]
                n213 = xnode "Opto out"("A/DIO9 (Pin 29)"=TRUE) -> ()  [unwired: 1 in, 1 out]
              }
              frame #1 {
                n214 = xnode "Opto out 2"("A/DIO9 (Pin 29)"=FALSE) -> ()  [unwired: 1 in, 1 out]
                n215 = Wait (ms)(milliseconds to wait=u32 77) -> ()  [unwired: 1 out]
              }
            }
          }
        }
        n216 = local read "Stop"() -> (w107:bool)
      }
    }
  }
